vi "Create Events.vi"(8 "error in (no error)":errorcluster, 11 "UserEvents in":refnum<class "User Events.lvclass">) -> (0 "error out":errorcluster, 3 "UserEvents out":refnum<class "User Events.lvclass">)   [LabVIEW 2016, in "User Events.lvclass"]
uses:
  User Events.lvclass
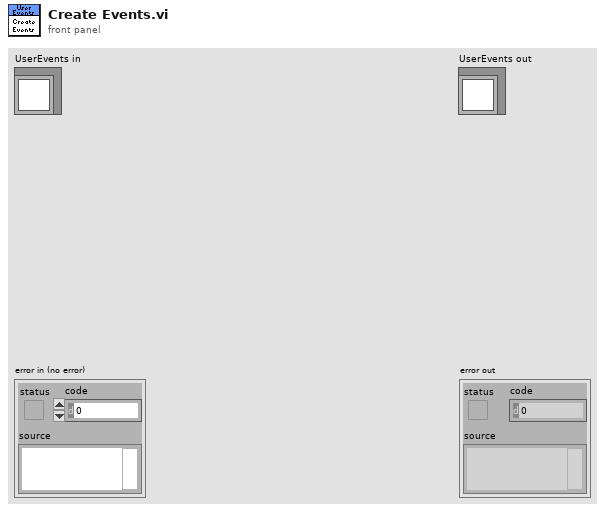
[diagram p1: front panel]
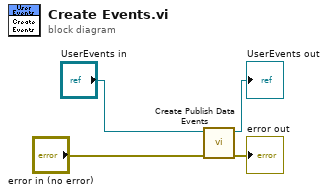
[diagram p0: block diagram]
diagram:
  n1 = call "Create Publish Data Events.vi"("error in (no error)"="error in (no error)", "UserEvents in"="UserEvents in") -> ("error out"=→"error out":errorcluster, "UserEvents out"=→"UserEvents out":refnum<class "User Events.lvclass">)  [unwired: 8 in]
